vi "Zero crossings VI.vi"(11 "Derivate":dbl[](graph)) -> (3 "Number of crossings":i32)   [LabVIEW 2010]
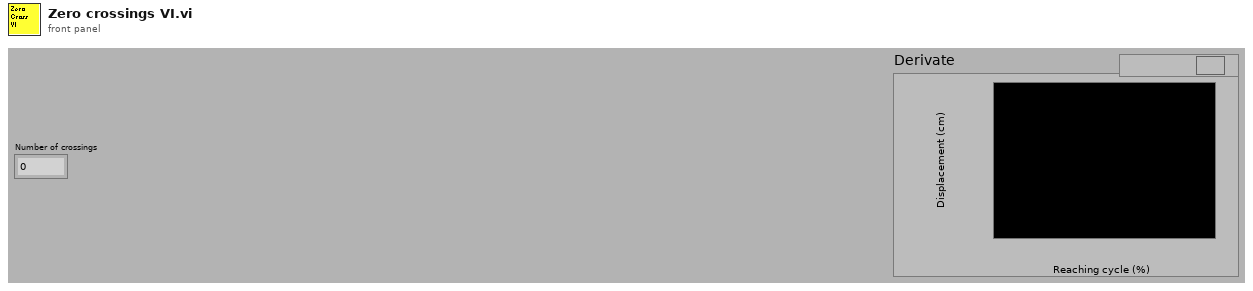
[diagram p1: front panel]
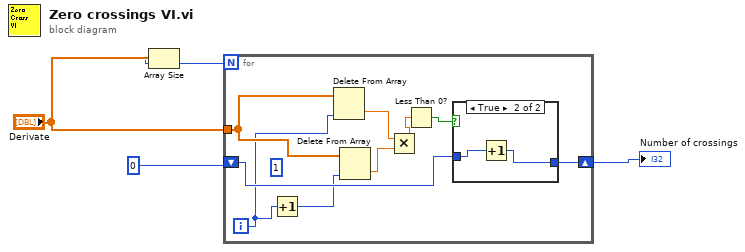
[diagram p0: block diagram]
diagram:
  n1 = Array Size(array="Derivate") -> (size(s)=w1:i32)
  n2 = for {
    N: w1 -> [_]
    shift-right: [w10] -> w3
    shift-left: 0 -> [w11]
    tunnel: "Derivate" -> [w8]
    i -> [w5]
    (unwired) 1
    n3 = Increment(x=w5) -> (x+1=w9:i32)
    n4 = Delete From Array(array=w8, index=w5) -> (deleted portion=w7:dbl)  [unwired: 1 in, 1 out]
    n5 = Delete From Array(array=w8, index=w9) -> (deleted portion=w6:dbl)  [unwired: 1 in, 1 out]
    n6 = Multiply(x=w7, y=w6) -> (x*y=w12:dbl)
    n7 = Less Than 0?(x=w12) -> (x < 0?=w13:bool)
    n8 = case shown="True" w13 {
      tunnel: w11 -> [w14 w15]
      tunnel: [w14 w16] -> w10
      frame False {
      }
      frame True {
        n9 = Increment(x=w15) -> (x+1=w16:i32)
      }
    }
  }
  "Number of crossings" <- w3
